vi "10.5 Reading and Analyzing Data.vi"() -> ()   [LabVIEW 2019]
uses:
  <vilib>/Utility/file.llb/Read Delimited Spreadsheet (DBL).vi
panel:
  out "Data in one String":string
  out "Data in 2D array":dbl[][](array[numeric])
  in  "File Path Control":path
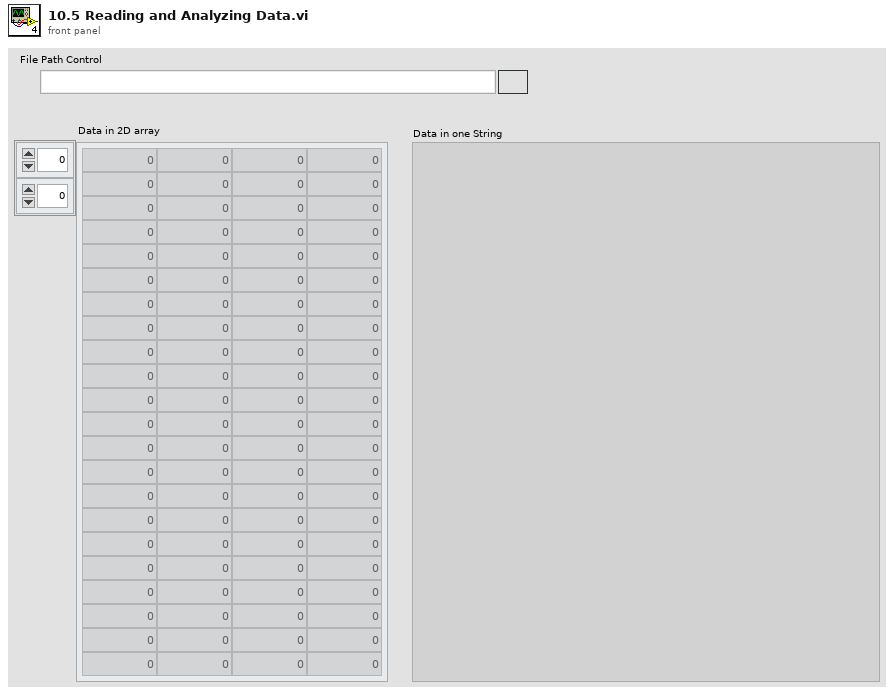
[diagram p1: front panel]
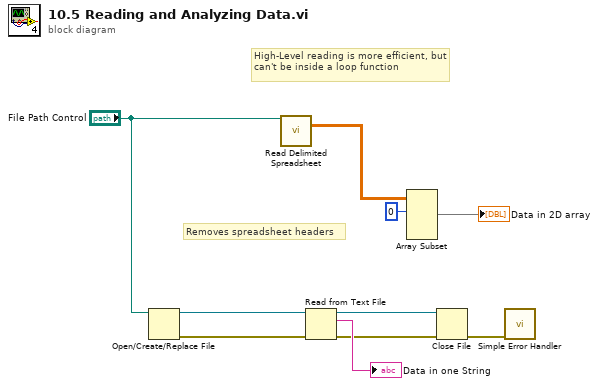
[diagram p0: block diagram]
diagram:
  # "High-Level reading is more efficient, but can't be inside a loop function"
  # "Removes spreadsheet headers"
  n1 = Open/Create/Replace File(file path (use dialog)="File Path Control") -> (refnum out=w6:refnum<file>, error out=w5:errorcluster)  [unwired: 5 in, 1 out]
  n2 = call-poly <vilib>:"Read Delimited Spreadsheet.vi"("file path (dialog if empty)"="File Path Control") -> ("all rows"=w10:dbl[][])  [unwired: 9 in, 5 out]
  n3 = Read from Text File(file (use dialog)=w6, error in=w5) -> (refnum out=w3:refnum<file>, text=→"Data in one String":string, error out=w2:errorcluster)  [unwired: 2 in, 1 out]
  n4 = Array Subset "Array Subset"(array=w10, index (row)=0 ("index")) -> (→"Data in 2D array":dbl[][])  [unwired: 3 in]
  n5 = Close File(refnum=w3, error in=w2) -> (error out=w1:errorcluster)  [unwired: 1 out]
  n6 = call <vilib>:"Simple Error Handler.vi"("error in (no error)"=w1) -> ()  [unwired: 4 in, 5 out]
